vi "SpectroscopicMeasurementsMainUI.vi"() -> ()   [LabVIEW 2017]
uses:
  Spectrometer Utilities/SpectrometerControllerEnum.ctl
  Scripts Actors/MapScriptGFVEnum.ctl
  Microscope/MicroscopeControllerEnum.ctl
  AEROTECstageAPI/StageEnum.ctl
  Database/DatabaseContollerGFVenum.ctl
  SpectroMeasurementCtrlEnum.ctl
  Scripts Actors/MapDryScriptGFVEnum.ctl
  AEROTECstageAPI/SingleStageData.ctl
  AEROTECstageAPI/MoveDistanceInAxis.ctl
  Utility/Axis Direction Definition.ctl
  <vilib>/vision/Image Controls.llb/IMAQ Image.ctl
panel:
  in  "Abort":bool=TRUE
  out "Emergency String":string
  in  "Setup":u16(ring) caption="Combo Box" items=["Gulliver", "Perlman"]
  in  "Add/Remove User":bool
  out "User Picture":T1(plugin-control)
  in  "User Name":u16(ring) caption="Combo Box" items=["Netanela Cohen", "Omer Yaffe", "Matan Menahem", "Roman Korobko", "Lior Segev", "Maor Asher"]
  in  "Script":u16(ring) caption="Combo Box" items=["Map", "Map(dry)"]
  in  "Home Button":bool
  in  "Enable Stage":bool
  out "Y":dbl format="%.2g µm"
  out "Stage":bool
  out "X":dbl format="%.2g µm"
  in  "Right Button":bool
  in  "Left Button":bool
  in  "Down Button":bool
  in  "Up Button":bool
  in  "Distance (mm)":i32(slide)=9 min=1 max=10 step=1 scale=1.0..10.0
  out "JournalTable":string[][](table)=[["1/1/2017 6:00:00 AM", "test 3"], ["1/1/2017 4:00:00 AM", "Test 2"], ["1/1/2017 2:00:00 AM", "This is a test"]]
  out "System Health Status":string
  # "Yaffe's Lab"
  # "Raman Spectrometer Software - Data Acquisition Software (Weizmann Institute of Science)"
  # "Includes icons made by Daniel Bruce (danielbruce.se)"
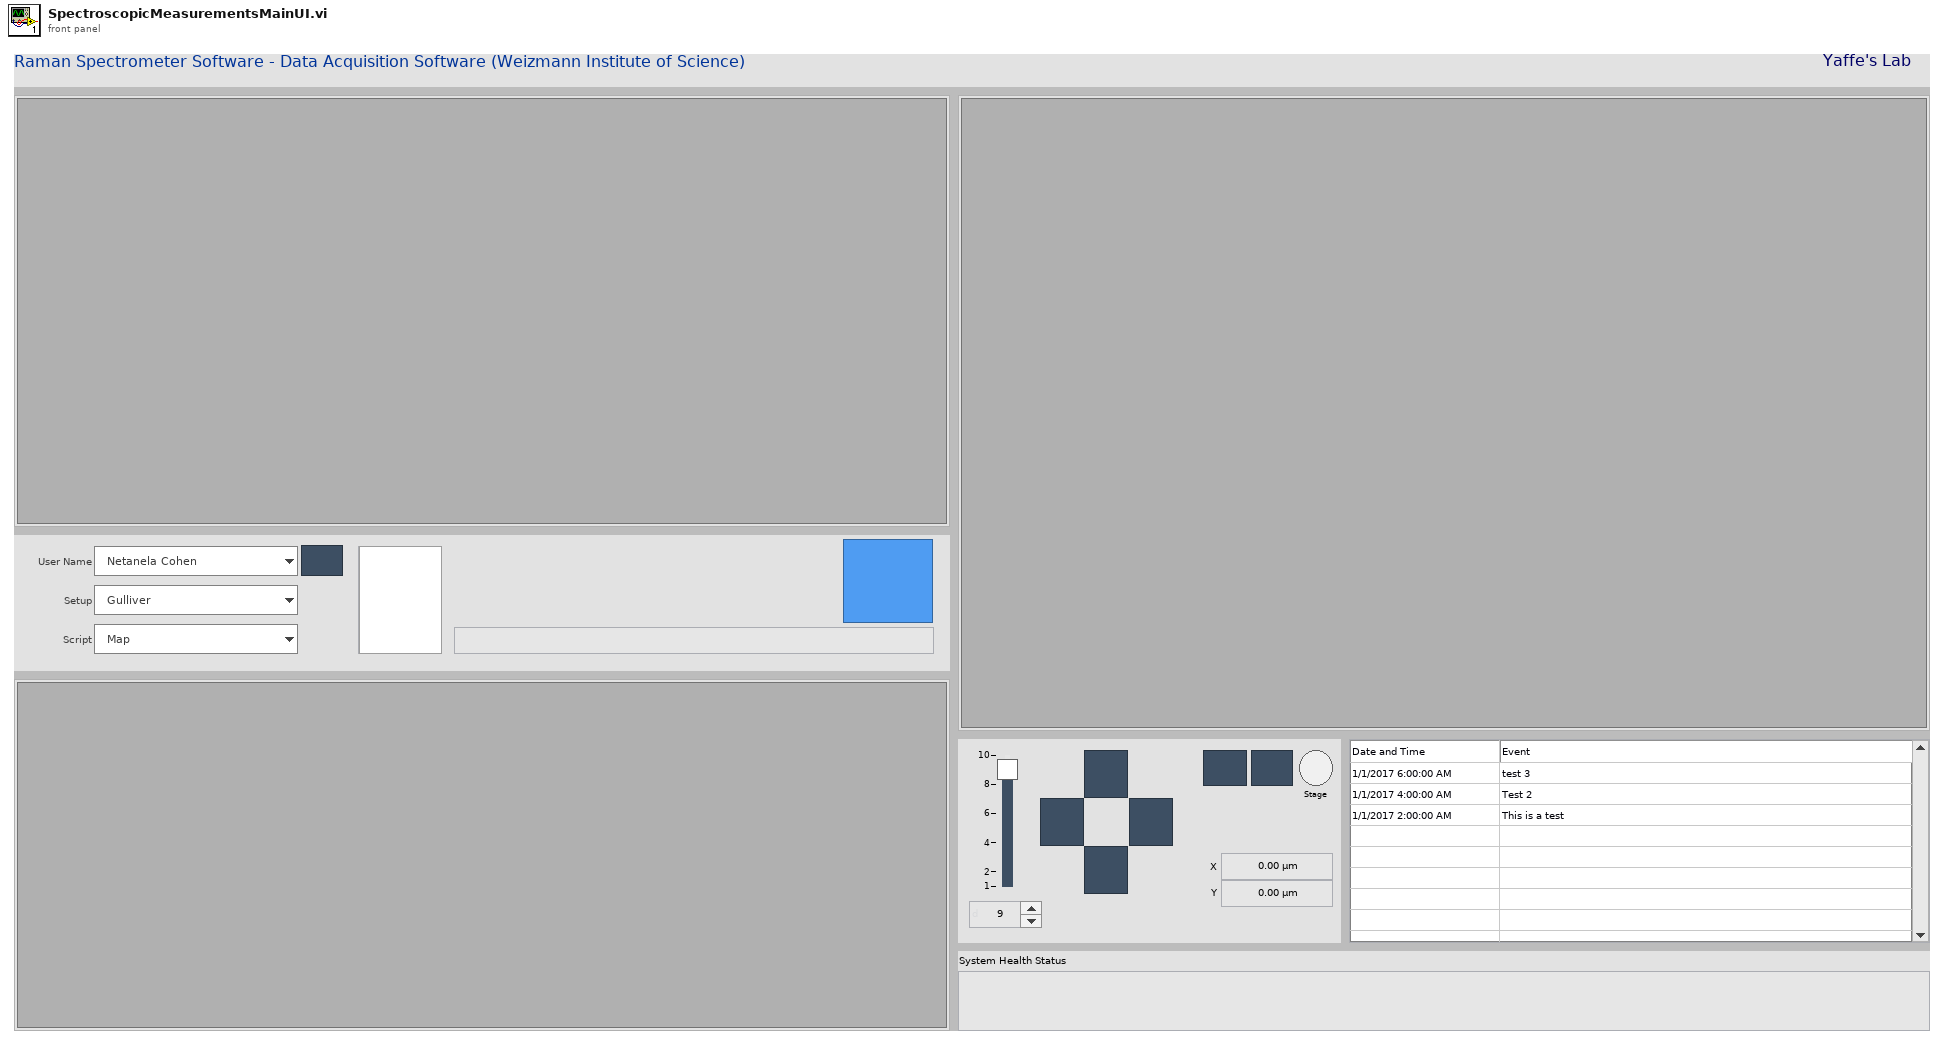
[diagram p1: front panel]
types:
  T1 = typedef "IMAQ Image.ctl" = refnum<image>
  T2 = typedef "SpectroMeasurementCtrlEnum.ctl" = enum16{"Init", "InsertMeasurementScript", "InsertSetupIndex", "InsertCurrentUserIndex", "GetAllData!"}
  T3 = typedef "DatabaseContollerGFVenum.ctl" = enum16{"Init and Open Database!", "GetTimeDifferencebetweenLastTwoMeasurements!", "Get next Journal Number!", "WriteInJournalTable", "GetNewMeas_dataIndex", "UpdateWithSpectrometerData", "UpdateWithMicroscopeData", "UpdateWithMapScriptData", "UpdateWithmainUIData", "Get Objective Microns/Pixels", "Get User Name!", "Get Active Users Names!", "Get User Picture!", "Get User Phone Number!", "Get Setup Names!", "Get Active Microscope Objectives!", "Get Experiment Number!", "Get Sample Types!", "Write meas_conf Table", "Write meas_data Table", "GetListOfIndices", "Get Objective Index", "Get last X Journal Entries"}
  T4 = typedef "StageEnum.ctl" = enum16{"Get Current Pos!", "Move axis!", "Enable Stage!", "Stop Stage Controller!", "Set Default Speeds!", "Get Stage Parameters", "Start Stage Controller!", "Init", "Go Home!"}
  T5 = typedef "SpectrometerControllerEnum.ctl" = enum16{"Init!", "Start!", "Stop!", "Start New Measurement!", "Update Current Measurement Data", "Set Current Measurement Ended Successfully", "Get Current Measurement Data!", "Get Current Measurement Ended Successfully", "GetSpectrometerVIRef!", "Insert Callback Event", "GetAllData!"}
  T6 = typedef "MicroscopeControllerEnum.ctl" = enum16{"GetAllData!", "Init!", "Start!", "Stop!", "GetMicroscopeVIRef", "CalculateRelPointForStagemicrons", "InsertCallbackEvent!", "InsertLaserPoint!", "InsertMapPoints!", "InsertMicroscopeOverlayImageRef!", "GetMicroscopeOverlayImageRef", "InsertObjectiveIndex!", "InsertLiveImageRef", "GetLiveImageRef"}
  T7 = typedef "MapScriptGFVEnum.ctl" = enum16{"GetAllData!", "InsertCoordData!", "InsertExperimentTitle", "Init!", "Stop!", "Start!", "GetMapScriptActorViRef", "InsertExperimentNumber", "InsertSampleType", "InsertMicroscopeImage"}
  T8 = typedef "SingleStageData.ctl" = cluster{"Desired Speed(mm/s)":dbl, "Desired Distance(mm)":dbl, "Enabled?":bool, "Moving?":bool, "Position(microns)":dbl}
  T9 = typedef "Axis Direction Definition.ctl" = enum16{"Axis left/right", "Axis up/down"}
  T10 = typedef "MoveDistanceInAxis.ctl" = cluster{"Axis Number":i16, "Distance (microns)":dbl}
  T11 = typedef "MapDryScriptGFVEnum.ctl" = enum16{"Init!", "Stop!", "Start!", "GetMapScriptActorViRef"}
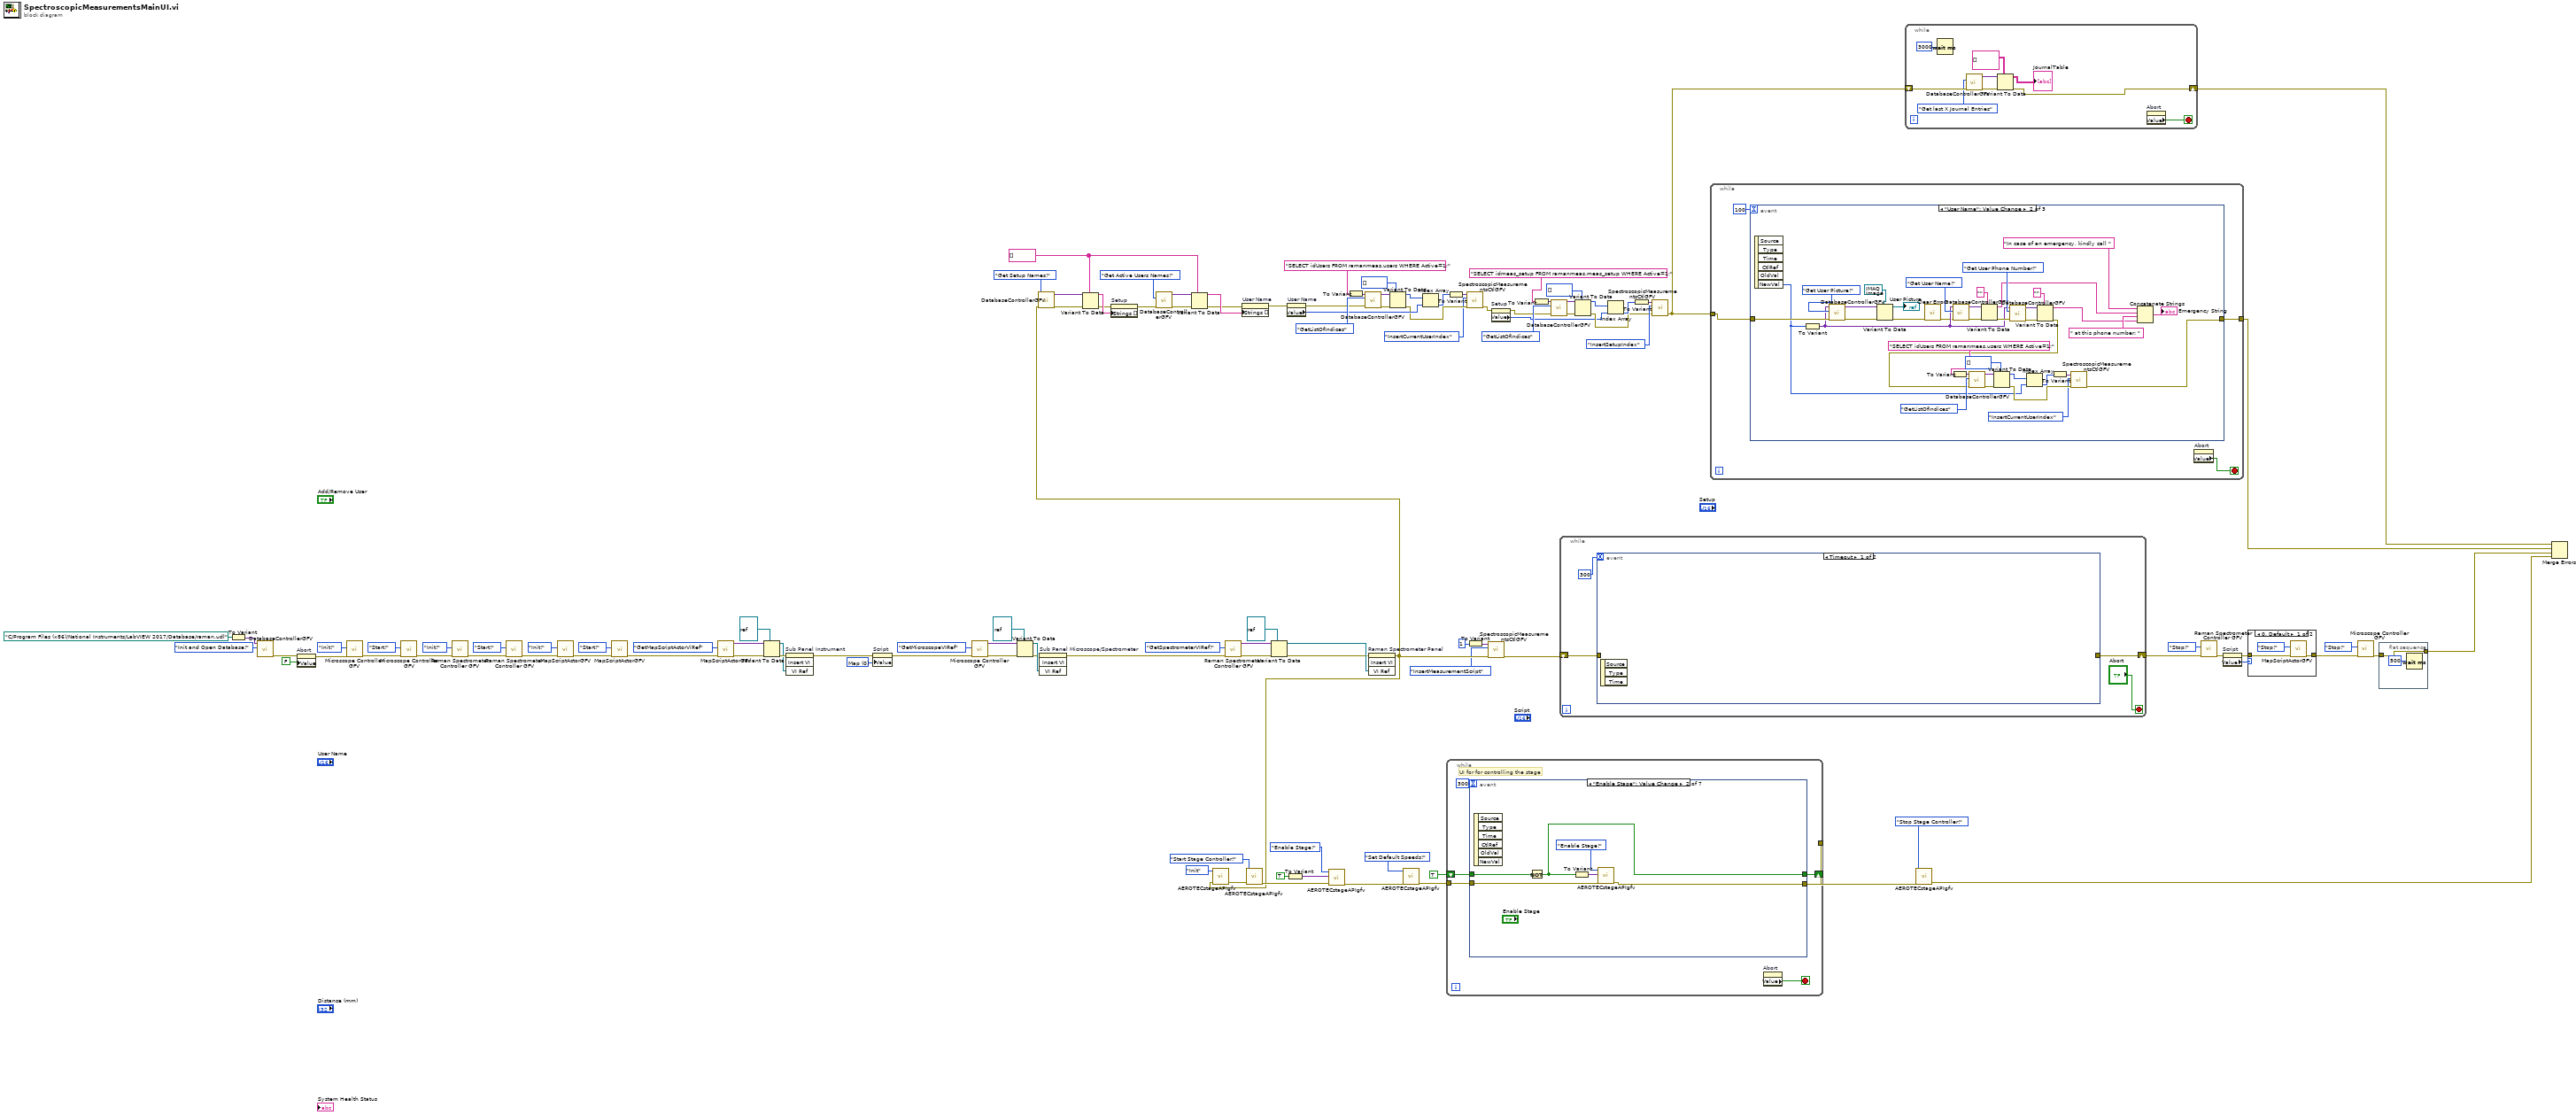
[diagram p0: block diagram]
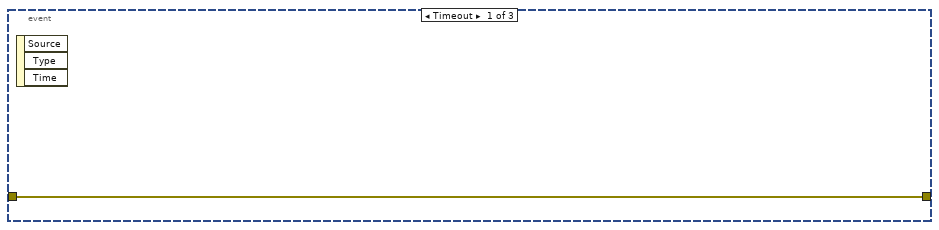
[diagram p2: hidden frame]
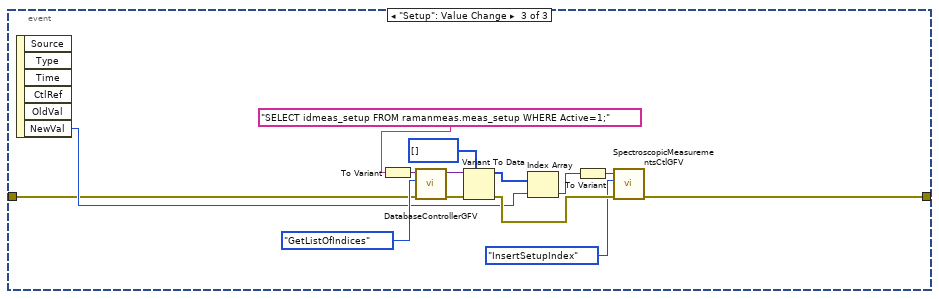
[diagram p3: hidden frame]
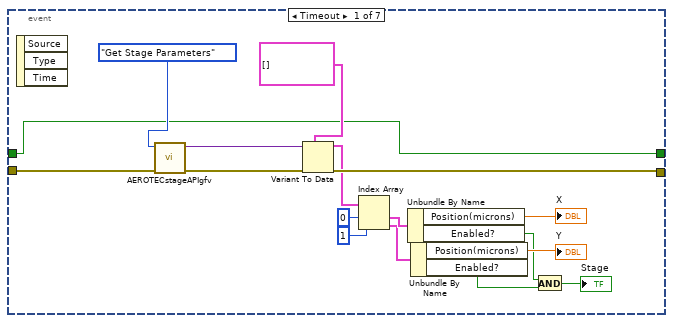
[diagram p4: hidden frame]
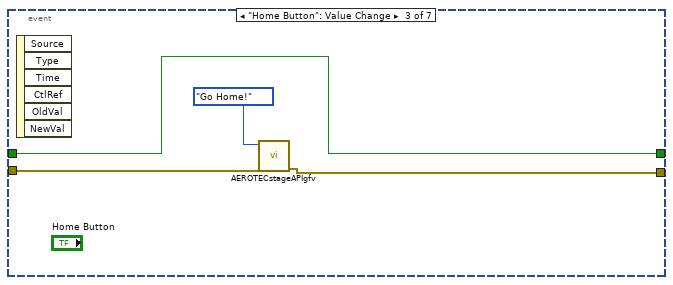
[diagram p5: hidden frame]
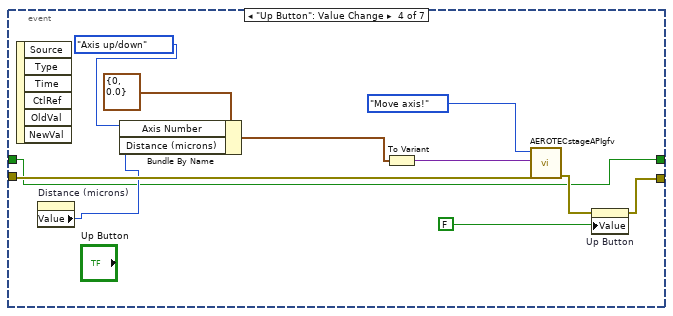
[diagram p6: hidden frame]
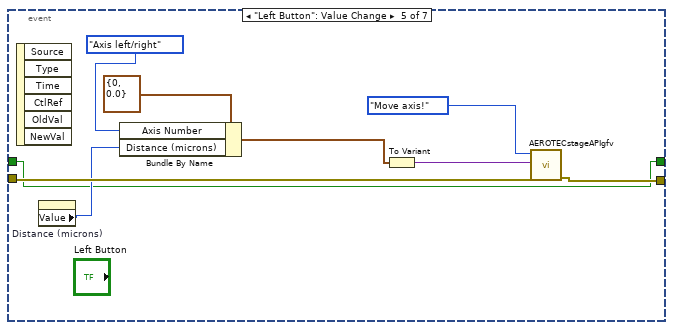
[diagram p7: hidden frame]
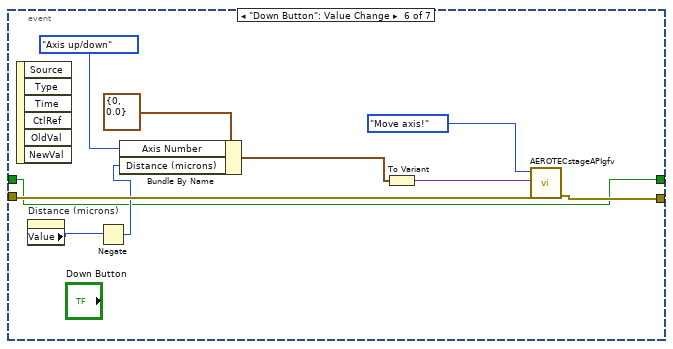
[diagram p8: hidden frame]
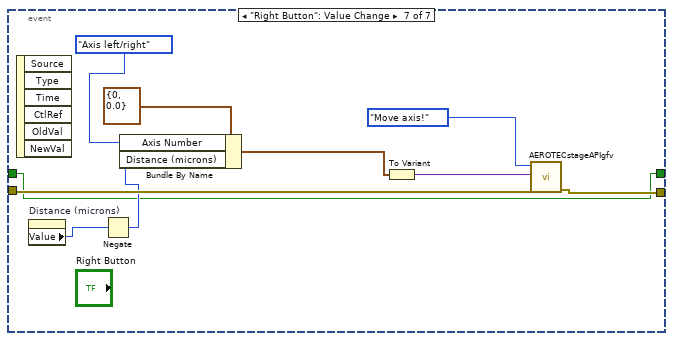
[diagram p9: hidden frame]
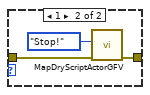
[diagram p10: hidden frame]
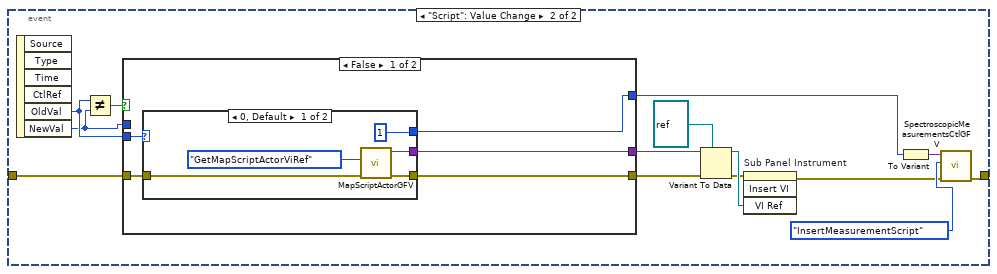
[diagram p11: hidden frame]
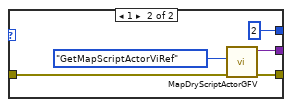
[diagram p12: hidden frame]
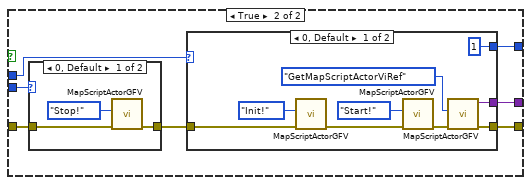
[diagram p13: hidden frame]
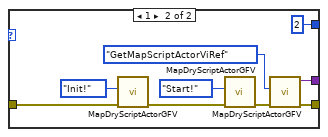
[diagram p14: hidden frame]
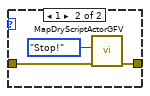
[diagram p15: hidden frame]
diagram:
  w40 = u16 0 items=["Map", "Map(dry)"] ("Script")
  w46 = string[] []
  n1 = To Variant(anything=path "C:/Program Files (x86)/National Instruments/LabVIEW 2017/Database/raman.udl" ("connection information")) -> (Variant=w56:variant)
  n2 = call "DatabaseControllerGFV.vi"("Enum"=DatabaseContollerGFVenum."Init and Open Database!", "Data in"=w56) -> ("error out"=w39:errorcluster)  [unwired: 8 in, 1 out]
  n3 = property on="Abort" class="Bool (strict)"(error in=w39, "Value"=FALSE ("stop")) -> (error out=w50:errorcluster)  [unwired: 1 in, 1 out]
  n4 = call "Microscope Controller GFV.vi"("error in (no error)"=w50, "MicroscopeEnum"=MicroscopeControllerEnum."Init!") -> ("error out"=w90:errorcluster)  [unwired: 8 in, 1 out]
  n5 = call "Microscope Controller GFV.vi"("error in (no error)"=w90, "MicroscopeEnum"=MicroscopeControllerEnum."Start!") -> ("error out"=w92:errorcluster)  [unwired: 8 in, 1 out]
  n6 = call "Raman Spectrometer Controller GFV.vi"("SpectrometerEnum"=SpectrometerControllerEnum."Init!", "error in (no error)"=w92) -> ("error out"=w111:errorcluster)  [unwired: 7 in, 1 out]
  n7 = call "Raman Spectrometer Controller GFV.vi"("SpectrometerEnum"=SpectrometerControllerEnum."Start!", "error in (no error)"=w111) -> ("error out"=w107:errorcluster)  [unwired: 7 in, 1 out]
  n8 = call "MapScriptActorGFV.vi"("error in (no error)"=w107, "MapScriptEnum"=MapScriptGFVEnum."Init!" ("Enum")) -> ("error out"=w105:errorcluster)  [unwired: 8 in, 1 out]
  n9 = call "MapScriptActorGFV.vi"("error in (no error)"=w105, "MapScriptEnum"=MapScriptGFVEnum."Start!" ("Enum")) -> ("error out"=w95:errorcluster)  [unwired: 8 in, 1 out]
  n10 = call "MapScriptActorGFV.vi"("error in (no error)"=w95, "MapScriptEnum"=MapScriptGFVEnum."GetMapScriptActorViRef") -> ("error out"=w94:errorcluster, "Data Out"=w93:variant)  [unwired: 8 in]
  n11 = Variant To Data(error in=w94, type=refnum<vi> refnum ("vi reference"), Variant=w93) -> (data=w97:refnum<vi>, error out=w98:errorcluster)
  n12 = invoke on="Sub Panel Instrument" class="SubPanel" method="Insert VI"(error in=w98, "VI Ref"=w97) -> (error out=w71:errorcluster)  [unwired: 2 in, 3 out]
  n13 = property on="Script" class="Ring (strict)"(error in=w71, "Value"=w40) -> (error out=w73:errorcluster)  [unwired: 1 in, 1 out]
  n14 = call "Microscope Controller GFV.vi"("error in (no error)"=w73, "MicroscopeEnum"=MicroscopeControllerEnum."GetMicroscopeVIRef") -> ("error out"=w84:errorcluster, "Data Out"=w83:variant)  [unwired: 8 in]
  n15 = Variant To Data(error in=w84, type=refnum<vi> refnum ("vi reference"), Variant=w83) -> (data=w82:refnum<vi>, error out=w81:errorcluster)
  n16 = invoke on="Sub Panel Microscope/Spectrometer" class="SubPanel" method="Insert VI"(error in=w81, "VI Ref"=w82) -> (error out=w72:errorcluster)  [unwired: 2 in, 3 out]
  n17 = call "Raman Spectrometer Controller GFV.vi"("SpectrometerEnum"=SpectrometerControllerEnum."GetSpectrometerVIRef!", "error in (no error)"=w72) -> ("Data Out"=w77:variant, "error out"=w78:errorcluster)  [unwired: 7 in]
  n18 = Variant To Data(error in=w78, type=refnum<vi> refnum ("vi reference"), Variant=w77) -> (data=w75:refnum<vi>, error out=w74:errorcluster)
  n19 = To Variant(anything=TRUE) -> (Variant=w63:variant)
  n20 = To Variant(anything="SELECT idUsers FROM ramanmeas.users WHERE Active=1;") -> (Variant=w38:variant)
  n21 = invoke on="Raman Spectrometer Panel" class="SubPanel" method="Insert VI"(error in=w74, "VI Ref"=w75) -> (error out=w10:errorcluster)  [unwired: 2 in, 3 out]
  n22 = call "DatabaseControllerGFV.vi"("error in (no error)"=w10, "Enum"=DatabaseContollerGFVenum."Get Setup Names!") -> ("error out"=w48:errorcluster, "Data Out"=w47:variant)  [unwired: 8 in]
  n23 = Variant To Data(error in=w48, type=w46, Variant=w47) -> (data=w44:string[], error out=w43:errorcluster)
  n24 = property on="Setup" class="Ring (strict)"(error in=w43, "Strings []"=w44) -> (error out=w42:errorcluster)  [unwired: 1 in, 1 out]
  n25 = call "DatabaseControllerGFV.vi"("error in (no error)"=w42, "Enum"=DatabaseContollerGFVenum."Get Active Users Names!") -> ("error out"=w54:errorcluster, "Data Out"=w53:variant)  [unwired: 8 in]
  n26 = Variant To Data(error in=w54, type=w46, Variant=w53) -> (data=w51:string[], error out=w41:errorcluster)
  n27 = call "AEROTECstageAPIgfv.vi"("error in (no error)"=w10, "StageContrlEnum"=StageEnum."Init") -> ("error out"=w69:errorcluster)  [unwired: 8 in, 1 out]
  n28 = property on="User Name" class="Ring (strict)"(error in=w41, "Strings []"=w51) -> (error out=w32:errorcluster)  [unwired: 1 in, 1 out]
  n29 = call "AEROTECstageAPIgfv.vi"("error in (no error)"=w69, "StageContrlEnum"=StageEnum."Start Stage Controller!") -> ("error out"=w60:errorcluster)  [unwired: 8 in, 1 out]
  n30 = property on="User Name" class="Ring (strict)"(error in=w32) -> (error out=w31:errorcluster, "Value"=w30:u16)  [unwired: 1 in, 1 out]
  n31 = call "AEROTECstageAPIgfv.vi"("error in (no error)"=w60, "Data in"=w63, "StageContrlEnum"=StageEnum."Enable Stage!") -> ("error out"=w59:errorcluster)  [unwired: 7 in, 1 out]
  n32 = call "DatabaseControllerGFV.vi"("error in (no error)"=w31, "Enum"=DatabaseContollerGFVenum."GetListOfIndices", "Data in"=w38) -> ("error out"=w35:errorcluster, "Data Out"=w34:variant)  [unwired: 7 in]
  n33 = Variant To Data(error in=w35, type=i32[] [], Variant=w34) -> (data=w29:i32[], error out=w28:errorcluster)
  n34 = call "AEROTECstageAPIgfv.vi"("error in (no error)"=w59, "StageContrlEnum"=StageEnum."Set Default Speeds!") -> ("error out"=w65:errorcluster)  [unwired: 8 in, 1 out]
  n35 = Index Array(array=w29, index=w30) -> (element=w26:i32)
  n36 = while {
    tunnel: w65 -> [w116]
    tunnel: [w115] -> w64
    shift-right: [w113] -> _
    shift-left: TRUE -> [w114]
    stop <- w112 stop-if-true
    # "UI for for controlling the stage"
    n37 = event shown="[1] \"Enable Stage\": Value Change" {
      selector: _ -> [_ _ _ _ _ _ _]
      dyn-events: _ -> [_ _ _ _ _ _ _]
      timeout: 300 -> [_ _ _ _ _ _ _]
      tunnel: w116 -> [w131 w139 w143 w154 w163 w173 w183]
      tunnel: [w129 w138 w142 w147 w162 w172 w182] -> w115
      tunnel: w114 -> [w118 w135 w140 w144 w155 w164 w174]
      tunnel: [w118 w134 w140 w144 w155 w164 w174] -> w113
      event Timeout {
        n38 = event-data() -> ()  [unwired: 1 in, 3 out]
        n39 = call "AEROTECstageAPIgfv.vi"("error in (no error)"=w131, "StageContrlEnum"=StageEnum."Get Stage Parameters") -> ("error out"=w129:errorcluster, "Data Out"=w133:variant)  [unwired: 8 in]
        n40 = Variant To Data(type=T8[] [], Variant=w133) -> (data=w128:T8[])  [unwired: 1 in, 1 out]
        n41 = Index Array(array=w128, index #1=0 ("index"), index #2=1 ("index")) -> (element #1=w125:T8, element #2=w124:T8)
        n42 = Unbundle By Name(w125) -> ("Position(microns)"=→"X":dbl, "Enabled?"=w120:bool)
        n43 = Unbundle By Name(w124) -> ("Position(microns)"=→"Y":dbl, "Enabled?"=w119:bool)
        n44 = And(x=w120, y=w119) -> (x .and. y?=→"Stage":bool)
      }
      event "Enable Stage": Value Change {
        n45 = event-data() -> ()  [unwired: 1 in, 6 out]
        n46 = Not(x=w135) -> (.not. x?=w134:bool)
        n47 = To Variant(anything=w134) -> (Variant=w136:variant)
        n48 = call "AEROTECstageAPIgfv.vi"("error in (no error)"=w139, "Data in"=w136, "StageContrlEnum"=StageEnum."Enable Stage!") -> ("error out"=w138:errorcluster)  [unwired: 7 in, 1 out]
      }
      event "Home Button": Value Change {
        n49 = event-data() -> ()  [unwired: 1 in, 6 out]
        n50 = call "AEROTECstageAPIgfv.vi"("error in (no error)"=w143, "StageContrlEnum"=StageEnum."Go Home!") -> ("error out"=w142:errorcluster)  [unwired: 8 in, 1 out]
      }
      event "Up Button": Value Change {
        n51 = event-data() -> ()  [unwired: 1 in, 6 out]
        n52 = property on="Distance (microns)" class="Slide (strict)"() -> ("Value"=w145:i32)  [unwired: 2 in, 2 out]
        n53 = Bundle By Name(cluster=T10 {"Axis Number"=0, "Distance (microns)"=0.0} ("MoveDistanceInAxis"), "Axis Number"=Axis_Direction_Definition."Axis up/down", "Distance (microns)"=w145) -> (w150:T10)
        n54 = To Variant(anything=w150) -> (Variant=w152:variant)
        n55 = call "AEROTECstageAPIgfv.vi"("error in (no error)"=w154, "Data in"=w152, "StageContrlEnum"=StageEnum."Move axis!") -> ("error out"=w148:errorcluster)  [unwired: 7 in, 1 out]
        n56 = property on="Up Button" class="Bool"(error in=w148, "Value"=FALSE ("Disable Stage")) -> (error out=w147:errorcluster)  [unwired: 1 in, 1 out]
      }
      event "Left Button": Value Change {
        n57 = event-data() -> ()  [unwired: 1 in, 6 out]
        n58 = property on="Distance (microns)" class="Slide (strict)"() -> ("Value"=w156:i32)  [unwired: 2 in, 2 out]
        n59 = Bundle By Name(cluster=T10 {"Axis Number"=0, "Distance (microns)"=0.0} ("MoveDistanceInAxis"), "Axis Number"=Axis_Direction_Definition."Axis left/right", "Distance (microns)"=w156) -> (w158:T10)
        n60 = To Variant(anything=w158) -> (Variant=w160:variant)
        n61 = call "AEROTECstageAPIgfv.vi"("error in (no error)"=w163, "Data in"=w160, "StageContrlEnum"=StageEnum."Move axis!") -> ("error out"=w162:errorcluster)  [unwired: 7 in, 1 out]
      }
      event "Down Button": Value Change {
        n62 = event-data() -> ()  [unwired: 1 in, 6 out]
        n63 = property on="Distance (microns)" class="Slide (strict)"() -> ("Value"=w165:i32)  [unwired: 2 in, 2 out]
        n64 = Negate(x=w165) -> (-x=w166:i32)
        n65 = Bundle By Name(cluster=T10 {"Axis Number"=0, "Distance (microns)"=0.0} ("MoveDistanceInAxis"), "Axis Number"=Axis_Direction_Definition."Axis up/down", "Distance (microns)"=w166) -> (w168:T10)
        n66 = To Variant(anything=w168) -> (Variant=w170:variant)
        n67 = call "AEROTECstageAPIgfv.vi"("error in (no error)"=w173, "Data in"=w170, "StageContrlEnum"=StageEnum."Move axis!") -> ("error out"=w172:errorcluster)  [unwired: 7 in, 1 out]
      }
      event "Right Button": Value Change {
        n68 = event-data() -> ()  [unwired: 1 in, 6 out]
        n69 = property on="Distance (microns)" class="Slide (strict)"() -> ("Value"=w175:i32)  [unwired: 2 in, 2 out]
        n70 = Negate(x=w175) -> (-x=w176:i32)
        n71 = Bundle By Name(cluster=T10 {"Axis Number"=0, "Distance (microns)"=0.0} ("MoveDistanceInAxis"), "Axis Number"=Axis_Direction_Definition."Axis left/right", "Distance (microns)"=w176) -> (w178:T10)
        n72 = To Variant(anything=w178) -> (Variant=w180:variant)
        n73 = call "AEROTECstageAPIgfv.vi"("error in (no error)"=w183, "Data in"=w180, "StageContrlEnum"=StageEnum."Move axis!") -> ("error out"=w182:errorcluster)  [unwired: 7 in, 1 out]
      }
    }
    n74 = property on="Abort" class="Bool (strict)"() -> ("Value"=w112:bool)  [unwired: 2 in, 2 out]
  }
  n75 = To Variant(anything=w26) -> (Variant=w25:variant)
  n76 = call "SpectroscopicMeasurementsCtlGFV.vi"("error in (no error)"=w28, "Enum"=SpectroMeasurementCtrlEnum."InsertCurrentUserIndex", "Data in"=w25) -> ("error out"=w13:errorcluster)  [unwired: 7 in, 1 out]
  n77 = To Variant(anything=u16 1 ("NewVal")) -> (Variant=w8:variant)
  n78 = call "SpectroscopicMeasurementsCtlGFV.vi"("error in (no error)"=w10, "Enum"=SpectroMeasurementCtrlEnum."InsertMeasurementScript", "Data in"=w8) -> ("error out"=w9:errorcluster)  [unwired: 7 in, 1 out]
  n79 = property on="Setup" class="Ring (strict)"(error in=w13) -> (error out=w12:errorcluster, "Value"=w11:u16)  [unwired: 1 in, 1 out]
  n80 = To Variant(anything="SELECT idmeas_setup FROM ramanmeas.meas_setup WHERE Active=1;") -> (Variant=w15:variant)
  n81 = call "DatabaseControllerGFV.vi"("error in (no error)"=w12, "Enum"=DatabaseContollerGFVenum."GetListOfIndices", "Data in"=w15) -> ("error out"=w17:errorcluster, "Data Out"=w18:variant)  [unwired: 7 in]
  n82 = while {
    shift-right: [w185] -> w103
    shift-left: w9 -> [w187]
    stop <- "Abort" stop-if-true
    n83 = event shown="[0] Timeout" {
      selector: _ -> [_ _]
      dyn-events: _ -> [_ _]
      timeout: 300 -> [_ _]
      tunnel: w187 -> [_ w201]
      tunnel: [_ w190] -> w185
      event Timeout {
        n84 = event-data() -> ()  [unwired: 1 in, 3 out]
      }
      event "Script": Value Change {
        n85 = event-data() -> ("OldVal"=w195:u16, "NewVal"=w194:u16)  [unwired: 1 in, 4 out]
        n86 = Not Equal?(x=w195, y=w194) -> (x != y?=w193:bool)
        n87 = case shown="False" w193 {
          tunnel: w201 -> [w205 w223]
          tunnel: [w203 w221] -> w197
          tunnel: [w204 w220] -> w196
          tunnel: w195 -> [w206 w219]
          tunnel: w194 -> [_ w218]
          tunnel: [w202 w217] -> w188
          frame False {
            n88 = case shown="0, Default" w206 {
              tunnel: [w211 w216] -> w204
              tunnel: [w209 w214] -> w203
              tunnel: w205 -> [w208 w213]
              tunnel: [u16 1 ("NewVal") u16 2 ("NewVal")] -> w202
              frame 0, Default {
                n89 = call "MapScriptActorGFV.vi"("error in (no error)"=w208, "MapScriptEnum"=MapScriptGFVEnum."GetMapScriptActorViRef") -> ("error out"=w211:errorcluster, "Data Out"=w209:variant)  [unwired: 8 in]
              }
              frame 1 {
                n90 = call "MapDryScriptActorGFV.vi"("error in (no error)"=w213, "MapScriptFGVEnum"=MapDryScriptGFVEnum."GetMapScriptActorViRef") -> ("error out"=w216:errorcluster, "Data Out"=w214:variant)  [unwired: 8 in]
              }
            }
          }
          frame True {
            n91 = case shown="0, Default" w219 {
              tunnel: w223 -> [w244 w246]
              tunnel: [w243 w247] -> w222
              frame 0, Default {
                n92 = call "MapScriptActorGFV.vi"("error in (no error)"=w244, "MapScriptEnum"=MapScriptGFVEnum."Stop!") -> ("error out"=w243:errorcluster)  [unwired: 8 in, 1 out]
              }
              frame 1 {
                n93 = call "MapDryScriptActorGFV.vi"("error in (no error)"=w246, "MapScriptFGVEnum"=MapDryScriptGFVEnum."Stop!") -> ("error out"=w247:errorcluster)  [unwired: 8 in, 1 out]
              }
            }
            n94 = case shown="0, Default" w218 {
              tunnel: w222 -> [w232 w241]
              tunnel: [w227 w236] -> w220
              tunnel: [w225 w234] -> w221
              tunnel: [u16 1 ("NewVal") u16 2 ("NewVal")] -> w217
              frame 0, Default {
                n95 = call "MapScriptActorGFV.vi"("error in (no error)"=w232, "MapScriptEnum"=MapScriptGFVEnum."Init!") -> ("error out"=w230:errorcluster)  [unwired: 8 in, 1 out]
                n96 = call "MapScriptActorGFV.vi"("error in (no error)"=w230, "MapScriptEnum"=MapScriptGFVEnum."Start!") -> ("error out"=w228:errorcluster)  [unwired: 8 in, 1 out]
                n97 = call "MapScriptActorGFV.vi"("error in (no error)"=w228, "MapScriptEnum"=MapScriptGFVEnum."GetMapScriptActorViRef") -> ("error out"=w227:errorcluster, "Data Out"=w225:variant)  [unwired: 8 in]
              }
              frame 1 {
                n98 = call "MapDryScriptActorGFV.vi"("error in (no error)"=w241, "MapScriptFGVEnum"=MapDryScriptGFVEnum."Init!") -> ("error out"=w239:errorcluster)  [unwired: 8 in, 1 out]
                n99 = call "MapDryScriptActorGFV.vi"("error in (no error)"=w239, "MapScriptFGVEnum"=MapDryScriptGFVEnum."Start!") -> ("error out"=w237:errorcluster)  [unwired: 8 in, 1 out]
                n100 = call "MapDryScriptActorGFV.vi"("error in (no error)"=w237, "MapScriptFGVEnum"=MapDryScriptGFVEnum."GetMapScriptActorViRef") -> ("error out"=w236:errorcluster, "Data Out"=w234:variant)  [unwired: 8 in]
              }
            }
          }
        }
        n101 = Variant To Data(error in=w196, type=refnum<vi> refnum ("vi reference"), Variant=w197) -> (data=w200:refnum<vi>, error out=w199:errorcluster)
        n102 = invoke on="Sub Panel Instrument" class="SubPanel" method="Insert VI"(error in=w199, "VI Ref"=w200) -> (error out=w189:errorcluster)  [unwired: 2 in, 3 out]
        n103 = To Variant(anything=w188) -> (Variant=w192:variant)
        n104 = call "SpectroscopicMeasurementsCtlGFV.vi"("error in (no error)"=w189, "Enum"=SpectroMeasurementCtrlEnum."InsertMeasurementScript", "Data in"=w192) -> ("error out"=w190:errorcluster)  [unwired: 7 in, 1 out]
      }
    }
  }
  n105 = Variant To Data(error in=w17, type=i32[] [], Variant=w18) -> (data=w20:i32[], error out=w21:errorcluster)
  n106 = Index Array(array=w20, index=w11) -> (element=w23:i32)
  n107 = To Variant(anything=w23) -> (Variant=w24:variant)
  n108 = call "SpectroscopicMeasurementsCtlGFV.vi"("error in (no error)"=w21, "Enum"=SpectroMeasurementCtrlEnum."InsertSetupIndex", "Data in"=w24) -> ("error out"=w2:errorcluster)  [unwired: 7 in, 1 out]
  n109 = while {
    tunnel: [w250] -> w5
    tunnel: w2 -> [w248]
    stop <- w249 stop-if-true
    n110 = event shown="[1] \"User Name\": Value Change" {
      selector: _ -> [_ _ _]
      dyn-events: _ -> [_ _ _]
      timeout: 100 -> [_ _ _]
      tunnel: w248 -> [w252 w285 w291]
      tunnel: [w252 w257 w290] -> w250
      event Timeout {
        n111 = event-data() -> ()  [unwired: 1 in, 3 out]
      }
      event "User Name": Value Change {
        n112 = event-data() -> ("NewVal"=w256:u16)  [unwired: 1 in, 5 out]
        n113 = To Variant(anything=w256) -> (Variant=w269:variant)
        n114 = call "DatabaseControllerGFV.vi"("error in (no error)"=w285, "Enum"=DatabaseContollerGFVenum."Get User Picture!", "Data in"=w269) -> ("error out"=w288:errorcluster, "Data Out"=w289:variant)  [unwired: 7 in]
        n115 = Variant To Data(error in=w288, type=T1 refnum ("Image Out"), Variant=w289) -> (data=→"User Picture":T1, error out=w254:errorcluster)
        n116 = call <vilib>:"Clear Errors.vi"("error in (no error)"=w254) -> ("error out"=w253:errorcluster)  [unwired: 5 in, 1 out]
        n117 = To Variant(anything="SELECT idUsers FROM ramanmeas.users WHERE Active=1;") -> (Variant=w268:variant)
        n118 = call "DatabaseControllerGFV.vi"("error in (no error)"=w253, "Enum"=DatabaseContollerGFVenum."Get User Name!", "Data in"=w269) -> ("error out"=w282:errorcluster, "Data Out"=w278:variant)  [unwired: 7 in]
        n119 = Variant To Data(error in=w282, type="", Variant=w278) -> (data=w272:string, error out=w281:errorcluster)
        n120 = call "DatabaseControllerGFV.vi"("error in (no error)"=w281, "Enum"=DatabaseContollerGFVenum."Get User Phone Number!", "Data in"=w269) -> ("error out"=w276:errorcluster, "Data Out"=w275:variant)  [unwired: 7 in]
        n121 = Variant To Data(error in=w276, type="", Variant=w275) -> (data=w270:string, error out=w255:errorcluster)
        n122 = call "DatabaseControllerGFV.vi"("error in (no error)"=w255, "Enum"=DatabaseContollerGFVenum."GetListOfIndices", "Data in"=w268) -> ("error out"=w267:errorcluster, "Data Out"=w266:variant)  [unwired: 7 in]
        n123 = Variant To Data(error in=w267, type=i32[] [], Variant=w266) -> (data=w265:i32[], error out=w264:errorcluster)
        n124 = Index Array(array=w265, index=w256) -> (element=w263:i32)
        n125 = To Variant(anything=w263) -> (Variant=w262:variant)
        n126 = call "SpectroscopicMeasurementsCtlGFV.vi"("error in (no error)"=w264, "Enum"=SpectroMeasurementCtrlEnum."InsertCurrentUserIndex", "Data in"=w262) -> ("error out"=w257:errorcluster)  [unwired: 7 in, 1 out]
        n127 = Concatenate Strings("In case of an emergency, kindly call ", w272, " at this phone number: ", w270) -> (→"Emergency String":string)
      }
      event "Setup": Value Change {
        n128 = event-data() -> ("NewVal"=w292:u16)  [unwired: 1 in, 5 out]
        n129 = To Variant(anything="SELECT idmeas_setup FROM ramanmeas.meas_setup WHERE Active=1;") -> (Variant=w297:variant)
        n130 = call "DatabaseControllerGFV.vi"("error in (no error)"=w291, "Enum"=DatabaseContollerGFVenum."GetListOfIndices", "Data in"=w297) -> ("error out"=w298:errorcluster, "Data Out"=w299:variant)  [unwired: 7 in]
        n131 = Variant To Data(error in=w298, type=i32[] [], Variant=w299) -> (data=w300:i32[], error out=w301:errorcluster)
        n132 = Index Array(array=w300, index=w292) -> (element=w302:i32)
        n133 = To Variant(anything=w302) -> (Variant=w303:variant)
        n134 = call "SpectroscopicMeasurementsCtlGFV.vi"("error in (no error)"=w301, "Enum"=SpectroMeasurementCtrlEnum."InsertSetupIndex", "Data in"=w303) -> ("error out"=w290:errorcluster)  [unwired: 7 in, 1 out]
      }
    }
    n135 = property on="Abort" class="Bool (strict)"() -> ("Value"=w249:bool)  [unwired: 2 in, 2 out]
  }
  n136 = while {
    shift-right: [w305] -> w1
    shift-left: w2 -> [w310]
    stop <- w311 stop-if-true
    n137 = Wait (ms)(milliseconds to wait=u32 3000) -> ()  [unwired: 1 out]
    n138 = call "DatabaseControllerGFV.vi"("error in (no error)"=w310, "Enum"=DatabaseContollerGFVenum."Get last X Journal Entries") -> ("error out"=w308:errorcluster, "Data Out"=w304:variant)  [unwired: 8 in]
    n139 = Variant To Data(error in=w308, type=string[][] [] ("JournalTable"), Variant=w304) -> (data=→"JournalTable":string[][], error out=w305:errorcluster)
    n140 = property on="Abort" class="Bool (strict)"() -> ("Value"=w311:bool)  [unwired: 2 in, 2 out]
  }
  n141 = call "AEROTECstageAPIgfv.vi"("error in (no error)"=w64, "StageContrlEnum"=StageEnum."Stop Stage Controller!") -> ("error out"=w4:errorcluster)  [unwired: 8 in, 1 out]
  n142 = call "Raman Spectrometer Controller GFV.vi"("SpectrometerEnum"=SpectrometerControllerEnum."Stop!", "error in (no error)"=w103) -> ("error out"=w101:errorcluster)  [unwired: 7 in, 1 out]
  n143 = property on="Script" class="Ring (strict)"(error in=w101) -> (error out=w100:errorcluster, "Value"=w102:u16)  [unwired: 1 in, 1 out]
  n144 = case shown="0, Default" w102 {
    tunnel: w100 -> [w315 w317]
    tunnel: [w314 w318] -> w88
    frame 0, Default {
      n145 = call "MapScriptActorGFV.vi"("error in (no error)"=w315, "MapScriptEnum"=MapScriptGFVEnum."Stop!") -> ("error out"=w314:errorcluster)  [unwired: 8 in, 1 out]
    }
    frame 1 {
      n146 = call "MapDryScriptActorGFV.vi"("error in (no error)"=w317, "MapScriptFGVEnum"=MapDryScriptGFVEnum."Stop!") -> ("error out"=w318:errorcluster)  [unwired: 8 in, 1 out]
    }
  }
  n147 = call "Microscope Controller GFV.vi"("error in (no error)"=w88, "MicroscopeEnum"=MicroscopeControllerEnum."Stop!") -> ("error out"=w87:errorcluster)  [unwired: 8 in, 1 out]
  n148 = flat-sequence {
    tunnel: w87 -> [w319]
    tunnel: [w319] -> _
    tunnel: [w319] -> w3
    frame #0 {
      n149 = Wait (ms)(milliseconds to wait=u32 500) -> ()  [unwired: 1 out]
    }
  }
  n150 = Merge Errors(w1, w5, w3, w4) -> ()  [unwired: 1 out]
